vi "Work.vi"(8 "error in (no error)":errorcluster, 9 "Outputs":refnum<class "Output.lvclass">[](array[class]), 10 "Inputs":refnum<class "Input.lvclass">[](array[class]), 11 "Block in":refnum<class "Block.lvclass">) -> (0 "error out":errorcluster, 3 "Block out":refnum<class "Block.lvclass">)   [LabVIEW 2020, in "Parallel Block.lvlib" / "Block.lvclass"]
uses:
  Block.lvclass
  Input/Input.lvclass
  Output/Output.lvclass
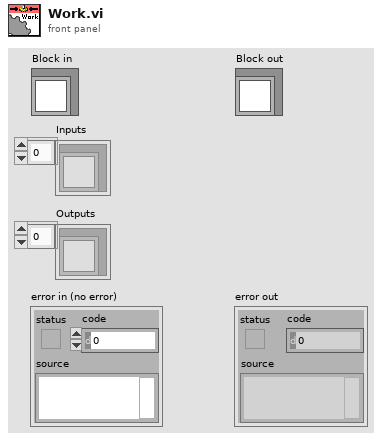
[diagram p1: front panel]
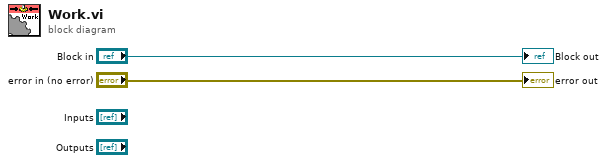
[diagram p0: block diagram]
diagram:
  "error out" <- "error in (no error)"
  "Block out" <- "Block in"
